vi "구구단_배열 만들기.vi"() -> ()   [LabVIEW 2020]
panel:
  out "배열 3":i32[][](array[numeric])
  out "출력 배열":i32[][](array[numeric])
  out "배열":i32[][](array[numeric])
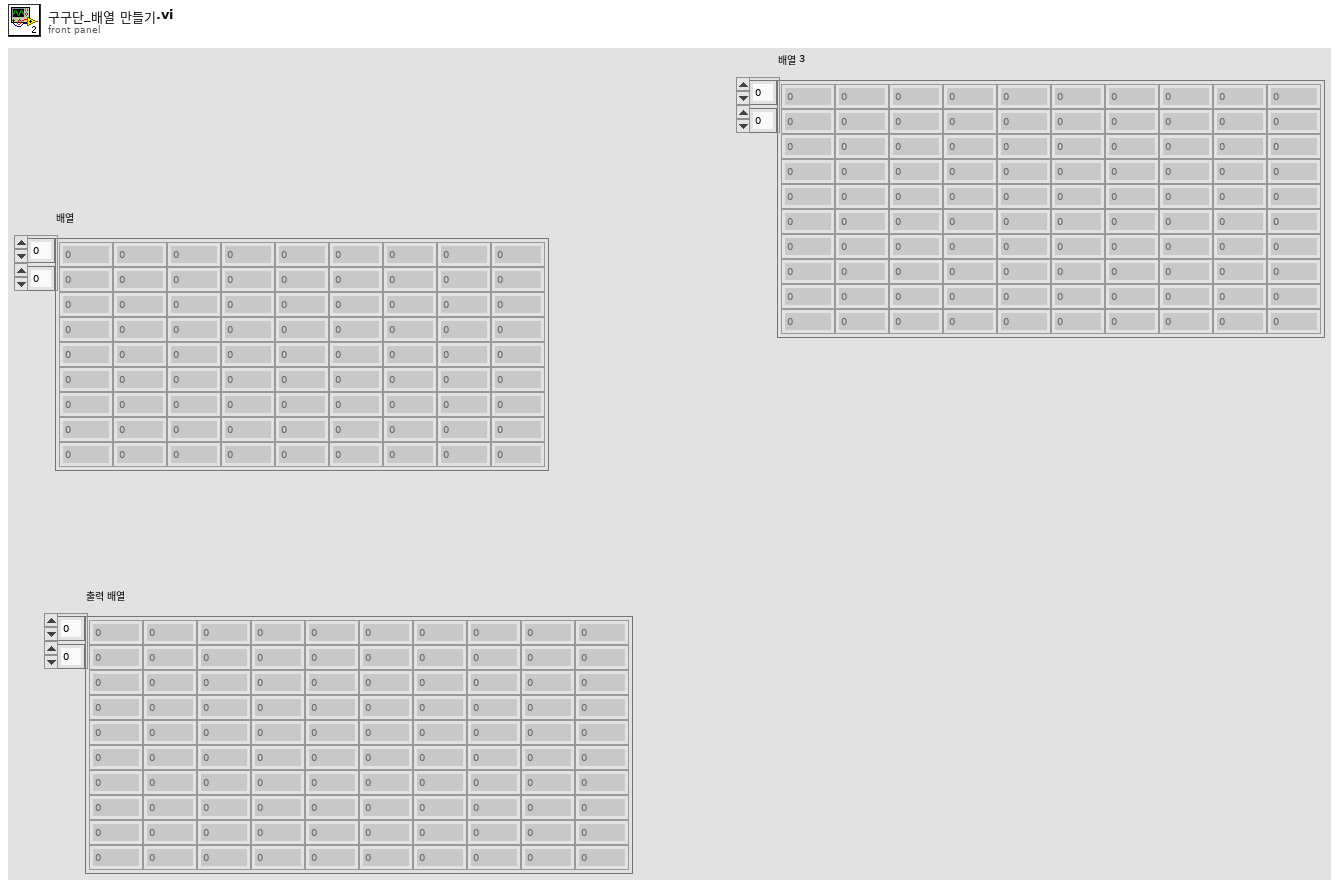
[diagram p1: front panel]
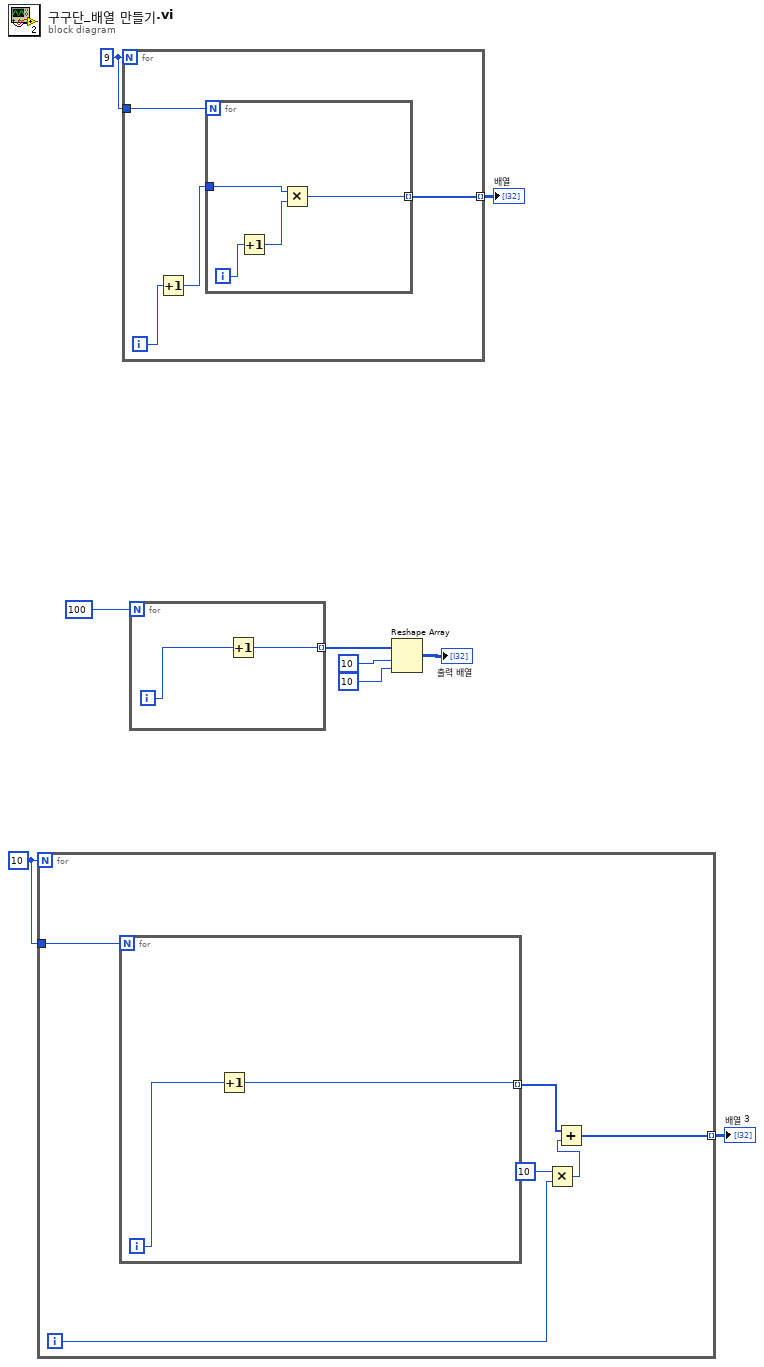
[diagram p0: block diagram]
diagram:
  w2 = 10
  w9 = 9
  n1 = for {
    N: w2 -> [_]
    tunnel: w2 -> [w15]
    tunnel: [w13] -> w1 mode=indexing
    i -> [w11]
    n2 = for {
      N: w15 -> [_]
      tunnel: [w17] -> w14 mode=indexing
      i -> [w16]
      n3 = Increment(x=w16) -> (x+1=w17:i32)
    }
    n4 = Multiply(x=10, y=w11) -> (x*y=w10:i32)
    n5 = Add(x=w14, y=w10) -> (x+y=w13:i32[])
  }
  "배열 3" <- w1
  n6 = for {
    N: w9 -> [_]
    tunnel: w9 -> [w21]
    tunnel: [w20] -> w8 mode=indexing
    i -> [w19]
    n7 = Increment(x=w19) -> (x+1=w18:i32)
    n8 = for {
      N: w21 -> [_]
      tunnel: w18 -> [w25]
      tunnel: [w24] -> w20 mode=indexing
      i -> [w23]
      n9 = Increment(x=w23) -> (x+1=w22:i32)
      n10 = Multiply(x=w25, y=w22) -> (x*y=w24:i32)
    }
  }
  "배열" <- w8
  n11 = for {
    N: 100 -> [_]
    tunnel: [w26] -> w6 mode=indexing
    i -> [w27]
    n12 = Increment(x=w27) -> (x+1=w26:i32)
  }
  n13 = Reshape Array(w6, 10 ("차원 크기"), 10 ("차원 크기")) -> (→"출력 배열":i32[][])
